vi "transmitter_6.vi"() -> ()   [LabVIEW 2022 SP3]
uses:
  <vilib>/addons/Modulation/Digital/General/MT Generate Bits (Galois, PN Order).vi
  <vilib>/addons/Modulation/Digital/Support/Common/Validators/mod_Generate Bits Validate.vi
  <vilib>/addons/Modulation/Analog/support/mod_Set Error Source.vi
  <vilib>/addons/Modulation/Digital/Support/Common/Validators/mod_AWGN Validate.vi
  <vilib>/addons/Modulation/Digital/Impairments/subVIs/mod_createSeeds.vi
  <vilib>/addons/Modulation/Digital/Support/Common/Validators/mod_Validate Samples Per Symbol.vi
  <vilib>/addons/Modulation/Analog/support/Validators/mod_Validate Complex Waveform.vi
  <vilib>/addons/Modulation/Analog/support/Validators/mod_WFErrorHandler.vi
  <vilib>/addons/Modulation/Digital/Support/Common/Validators/mod_Generate Filter Coefficients Validate.vi
  <vilib>/addons/Modulation/Digital/General/subVIs/mod_Generate Filter Coefficients.vi
  <vilib>/addons/Modulation/Digital/General/subVIs/mod_Generate Bits PN Sequence.vi
  <vilib>/addons/Modulation/Digital/General/MT Generate QAM System Parameters(M).vi
  <vilib>/Analysis/1siggen.llb/Gaussian White Noise (obs 90).vi
  <instrlib>/niUSRP/niUSRP Write Tx Data (CDB Cluster).vi
  <vilib>/addons/Modulation/niDMT.lvlib
  <vilib>/addons/Modulation/niAMT.lvlib
panel:
  in  "M-QAM (16)":i32=16
  in  "active antenna":string
  in  "device names":refnum<k15>
  in  "carrier frequency":dbl=100000.0 format="%#_6p"
  in  "gain":dbl format="%#_6f"
  in  "IQ rate":dbl=100000.0 format="%#_6p"
  in  "Eb/N0 (10 dB)":dbl=10.0
  in  "stop":bool
  out "Transmitted":T1(graph)
  out "Waveform Graph 2":waveform(dbl)(graph)
  out "Waveform Graph":waveform(dbl)(graph)
  in  "total bits (128)":i32=128
  out "bits per symbol":i32
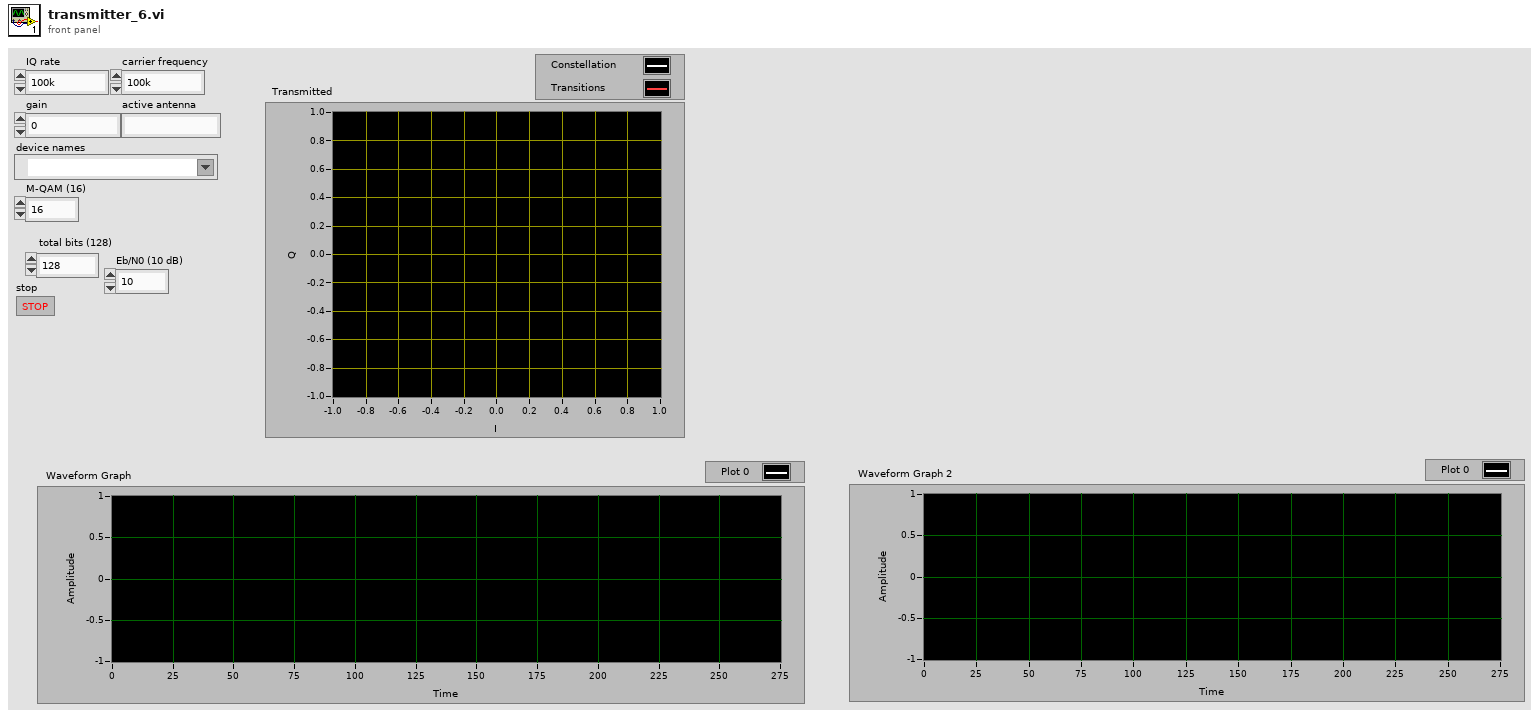
[diagram p1: front panel]
types:
  T1 = cluster{"Decimated Array":dbl[], "Decimated Array":dbl[]}[]
  T2 = enum16{"none", "Raised Cosine", "Root Raised Cos", "Gaussian"}
  T3 = enum16{"FSK", "PSK", "QAM", "MSK", "PAM", "ASK", "CPM"}
  T4 = cluster{"samples per symbol (16)":i32, "symbol map":cdb[]}
  T5 = typedef "niAMT.lvlib/Complex Data Waveform.ctl" = cluster{"t0":dbl, "dt":dbl, "Y":cdb[]}
  T6 = cluster{"constellation":dbl[], "oversampled data":dbl[]}[]
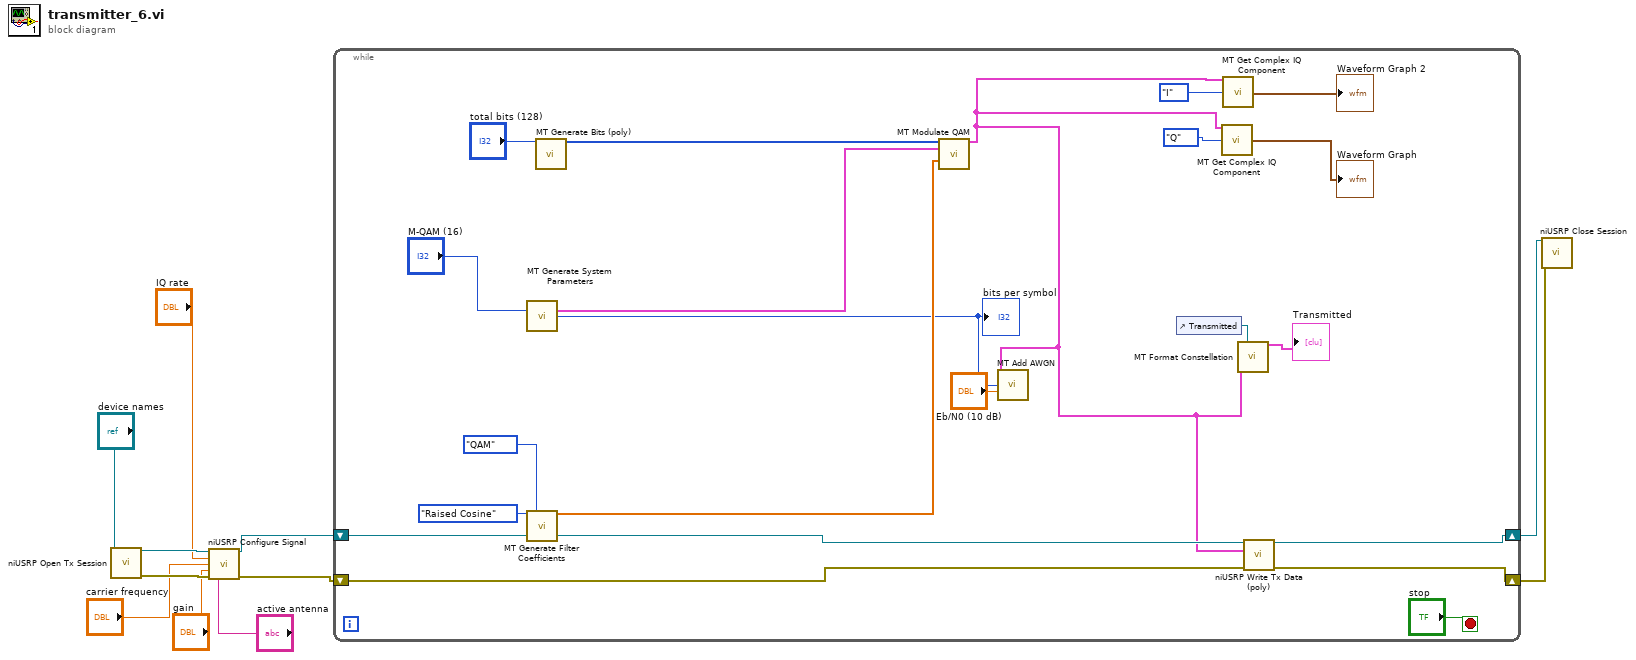
[diagram p0: block diagram]
diagram:
  n1 = call <instrlib>:"niUSRP Open Tx Session.vi"("device names"="device names") -> ("session handle out"=w11:refnum<k15>, "error out"=w10:errorcluster)  [unwired: 13 in]
  n2 = call <instrlib>:"niUSRP Configure Signal.vi"("session handle"=w11, "IQ rate"="IQ rate", "carrier frequency"="carrier frequency", "gain"="gain", "error in (no error)"=w10, "active antenna"="active antenna") -> ("session handle out"=w9:refnum<k15>, "error out"=w8:errorcluster)  [unwired: 5 in, 3 out]
  n3 = while {
    shift-right: [w16] -> w7
    shift-left: w9 -> [w18]
    shift-right: [w15] -> w6
    shift-left: w8 -> [w17]
    stop <- "stop" stop-if-true
    n4 = call-poly <vilib>:"MT Generate System Parameters.vi"("M-QAM (16)"="M-QAM (16)") -> ("QAM system parameters"=w32:T4, "bits per symbol"=w20:i32)  [unwired: 12 in, 1 out]
    "bits per symbol" <- w20
    n5 = call <vilib>:"MT Generate Filter Coefficients.vi"("pulse shaping filter (none)"=T2."Raised Cosine", "modulation type"=T3."QAM") -> ("pulse shaping filter coefficients"=w30:dbl[])  [unwired: 11 in, 2 out]
    n6 = call-poly <vilib>:"MT Generate Bits (poly).vi"("total bits (128)"="total bits (128)") -> ("output bit stream"=w31:i8[])  [unwired: 12 in, 2 out]
    n7 = call <vilib>:"MT Modulate QAM.vi"("input bit stream"=w31, "QAM system parameters"=w32, "pulse shaping filter coefficients"=w30) -> ("output complex waveform"=w13:T5)  [unwired: 10 in, 2 out]
    n8 = call <vilib>:"MT Add AWGN.vi"("input complex waveform"=w13, "bits per symbol (1)"=w20, "Eb/N0 (10 dB)"="Eb/N0 (10 dB)") -> ()  [unwired: 10 in, 3 out]
    n9 = control-ref of="Transmitted"() -> (w22:refnum<vi>)
    n10 = call <vilib>:"MT Get Complex IQ Component.vi"("IQ data (complex) in"=w13, "component choice"=enum16{"I", "Q", "Magnitude", "Phase"}."Q") -> ("CE component"=→"Waveform Graph":waveform(dbl))  [unwired: 11 in, 2 out]
    n11 = call <vilib>:"MT Get Complex IQ Component.vi"("IQ data (complex) in"=w13, "component choice"=enum16{"I", "Q", "Magnitude", "Phase"}."I") -> ("CE component"=→"Waveform Graph 2":waveform(dbl))  [unwired: 11 in, 2 out]
    n12 = call <vilib>:"MT Format Constellation.vi"("waveform"=w13, "constellation reference"=w22) -> ("constellation graph"=→"Transmitted":T6)  [unwired: 3 in, 10 out]
    n13 = call-poly <instrlib>:"niUSRP Write Tx Data (poly).vi"("session handle"=w18, "data"=w13, "error in (no error)"=w17) -> ("session handle out"=w16:refnum<k15>, "error out"=w15:errorcluster)  [unwired: 11 in]
  }
  n14 = call <instrlib>:"niUSRP Close Session.vi"("session handle"=w7, "error in (no error)"=w6) -> ()  [unwired: 13 in, 1 out]
